vi "Color_DrawOrange.vi"(9 "Expression":string, 11 "String in":refnum<vi>) -> (3 "String out":refnum<vi>)   [LabVIEW 2022 SP3]
uses:
  Color_Globals.vi
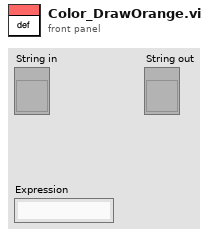
[diagram p1: front panel]
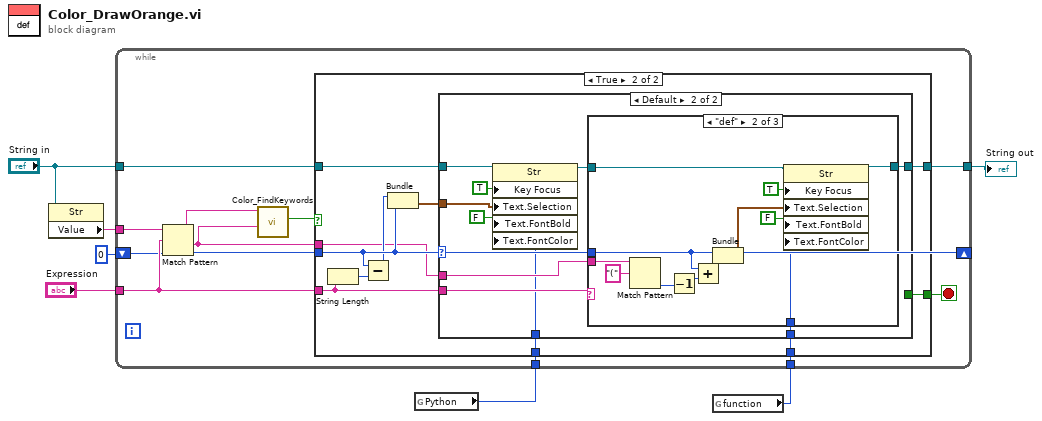
[diagram p0: block diagram]
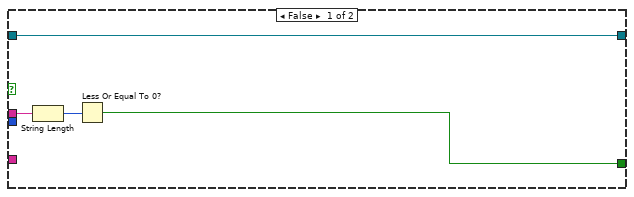
[diagram p2: hidden frame]
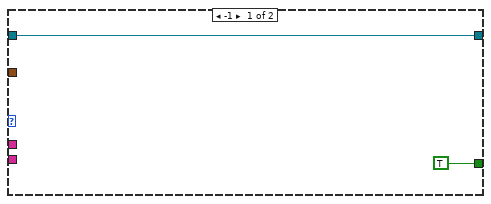
[diagram p3: hidden frame]
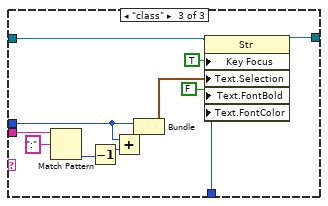
[diagram p5: hidden frame]
diagram:
  n1 = property on="Property Node" class="Str"(reference="String in") -> ("Value"=w3:string)  [unwired: 1 in, 2 out]
  n2 = global read "Color_Globals.vi" "Python"() -> (w1:u32)
  n3 = global read "Color_Globals.vi" "function"() -> (w2:u32)
  n4 = while {
    tunnel: "String in" -> [w19]
    shift-right: [w17] -> _
    shift-left: 0 -> [w12]
    tunnel: w3 -> [w13]
    tunnel: [w18] -> w6
    tunnel: "Expression" -> [w15]
    tunnel: w2 -> [w9]
    tunnel: w1 -> [w8]
    stop <- w16 stop-if-true
    n5 = Match Pattern(string=w13, regular expression=w15, offset (0)=w12) -> (before substring=w11:string, after substring=w14:string, offset past match=w17:i32)  [unwired: 1 out]
    n6 = call "Color_FindKeywords.vi"("After"=w14, "Before"=w11) -> ("Cmd?"=w10:bool)  [unwired: 9 in]
    n7 = case shown="True" w10 {
      tunnel: w19 -> [w23 w34]
      tunnel: [w23 w30] -> w18
      tunnel: w17 -> [_ w29]
      tunnel: [w20 w28] -> w16
      tunnel: w15 -> [_ w27]
      tunnel: w14 -> [w22 w26]
      tunnel: w9 -> [_ w25]
      tunnel: w8 -> [_ w24]
      frame False {
        n8 = String Length(string=w22) -> (length=w21:i32)
        n9 = Less Or Equal To 0?(x=w21) -> (x <= 0?=w20:bool)
      }
      frame True {
        n10 = String Length(string=w27) -> (length=w33:i32)
        n11 = Subtract(x=w29, y=w33) -> (x-y=w32:i32)
        n12 = Bundle(w32, "offset past match"=w29) -> (w31:cluster{i32, "offset past match":i32})  [unwired: 1 in]
        n13 = case shown="Default" w29 {
          selector: w29 -> [_ w41]
          tunnel: w34 -> [w36 w45]
          tunnel: w31 -> [_ w44]
          tunnel: [w36 w42] -> w30
          tunnel: [TRUE _] -> w28
          tunnel: w27 -> [_ w40]
          tunnel: w26 -> [_ w39]
          tunnel: w25 -> [_ w38]
          tunnel: w24 -> [_ w37]
          frame -1 {
          }
          frame Default {
            n14 = property on="Property Node" class="Str"(reference=w45, "Key Focus"=TRUE, "Text.Selection"=w44, "Text.FontBold"=FALSE ("Text.Font:Bold"), "Text.FontColor"=w37) -> (reference out=w43:refnum<vi>)  [unwired: 1 in, 1 out]
            n15 = case shown="\"def\"" w40 {
              tunnel: w43 -> [w48 w58 w70]
              tunnel: [w48 w57 w69] -> w42
              tunnel: w41 -> [_ w54 w66]
              tunnel: w39 -> [_ w52 w64]
              tunnel: w38 -> [_ w49 w61]
              frame Default {
              }
              frame "def" {
                n16 = Match Pattern(string=w52, regular expression="(") -> (offset past match=w50:i32)  [unwired: 1 in, 3 out]
                n17 = Decrement(x=w50) -> (x-1=w55:i32)
                n18 = Add(x=w54, y=w55) -> (x+y=w53:i32)
                n19 = Bundle("offset past match"=w54, w53) -> (w56:cluster{"offset past match":i32, i32})  [unwired: 1 in]
                n20 = property on="Property Node" class="Str"(reference=w58, "Key Focus"=TRUE, "Text.Selection"=w56, "Text.FontBold"=FALSE ("Text.Font:Bold"), "Text.FontColor"=w49) -> (reference out=w57:refnum<vi>)  [unwired: 1 in, 1 out]
              }
              frame "class" {
                n21 = Match Pattern(string=w64, regular expression=":") -> (offset past match=w62:i32)  [unwired: 1 in, 3 out]
                n22 = Decrement(x=w62) -> (x-1=w67:i32)
                n23 = Add(x=w66, y=w67) -> (x+y=w65:i32)
                n24 = Bundle("offset past match"=w66, w65) -> (w68:cluster{"offset past match":i32, i32})  [unwired: 1 in]
                n25 = property on="Property Node" class="Str"(reference=w70, "Key Focus"=TRUE, "Text.Selection"=w68, "Text.FontBold"=FALSE ("Text.Font:Bold"), "Text.FontColor"=w61) -> (reference out=w69:refnum<vi>)  [unwired: 1 in, 1 out]
              }
            }
          }
        }
      }
    }
  }
  "String out" <- w6
